vi "OldFieldToOOField.vi"(4 "Defense stretch":i32=500, 6 "Defense width":i32=1000, 8 "error in (no error)":errorcluster, 10 "geometry":T1, 11 "Field in":refnum<class "Field.lvclass">) -> (0 "error out":errorcluster, 3 "Field out":refnum<class "Field.lvclass">)   [LabVIEW 2023, in "Field.lvclass"]
uses:
  Field.lvclass
  Vision_class/Old vision/SSL Detection Frame Simple Estimator Cameras VelCmd Folder/Core/Field Size.ctl
  Field.lvclass/Field.ctl
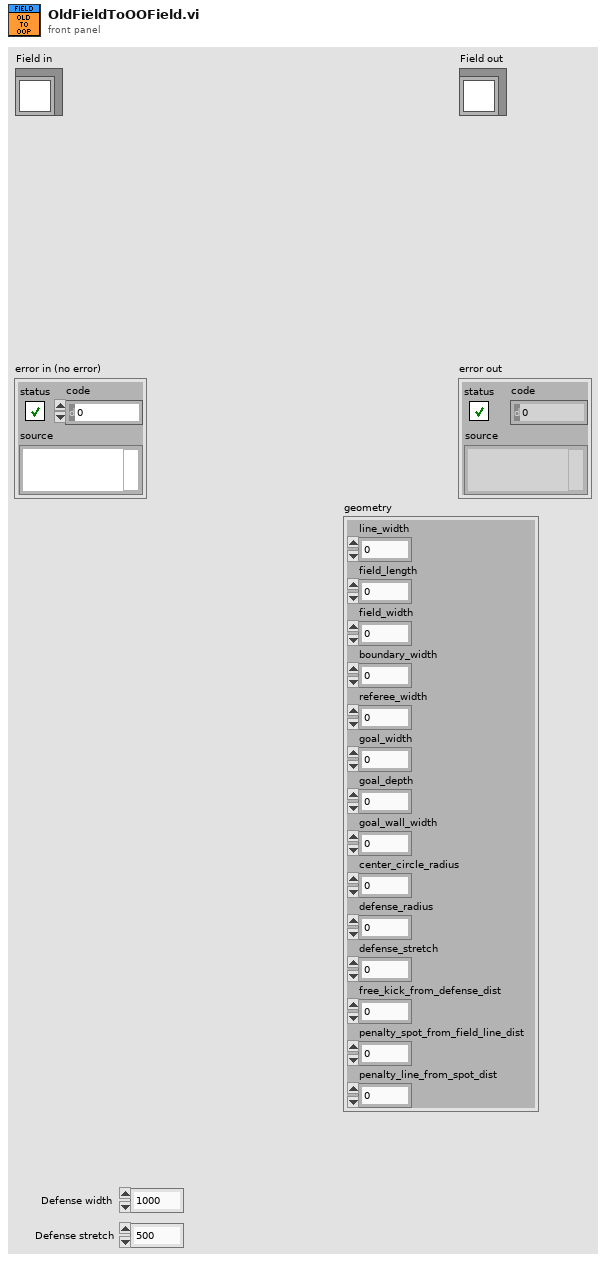
[diagram p1: front panel]
types:
  T1 = typedef "Field Size.ctl" = cluster{"line_width":u32, "field_length":u32, "field_width":u32, "boundary_width":u32, "referee_width":u32, "goal_width":u32, "goal_depth":u32, "goal_wall_width":u32, "center_circle_radius":u32, "defense_radius":u32, "defense_stretch":u32, "free_kick_from_defense_dist":u32, "penalty_spot_from_field_line_dist":u32, "penalty_line_from_spot_dist":u32}
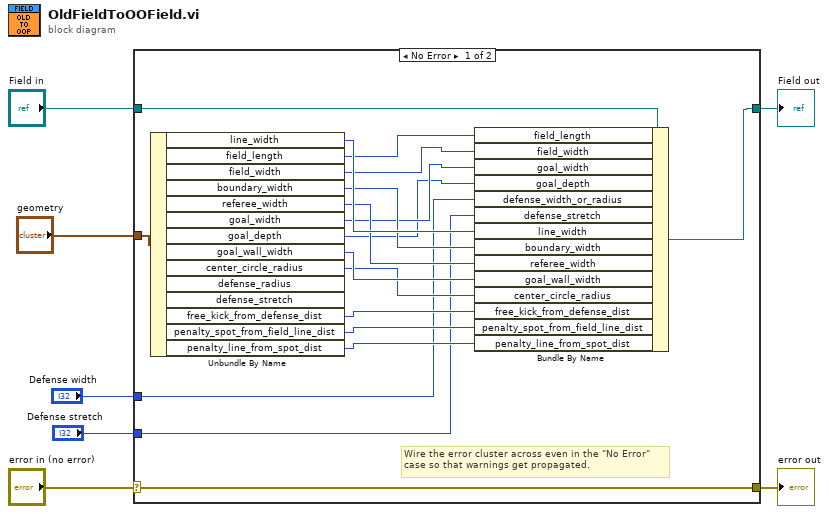
[diagram p0: block diagram]
diagram:
  n1 = case shown="No Error" "error in (no error)" {
    selector: "error in (no error)" -> [w25 w27]
    tunnel: [w25 w27] -> w6
    tunnel: [w10 w26] -> w4
    tunnel: "Field in" -> [w24 w26]
    tunnel: "geometry" -> [w23 _]
    tunnel: "Defense width" -> [w9 _]
    tunnel: "Defense stretch" -> [w8 _]
    frame No Error {
      # "Wire the error cluster across even in the \"No Error\"\ncase so that warnings get propagated."
      n2 = Unbundle By Name(w23) -> ("line_width"=w22:u32, "field_length"=w21:u32, "field_width"=w20:u32, "boundary_width"=w19:u32, "referee_width"=w18:u32, "goal_width"=w17:u32, "goal_depth"=w16:u32, "goal_wall_width"=w15:u32, "center_circle_radius"=w14:u32, "free_kick_from_defense_dist"=w13:u32, "penalty_spot_from_field_line_dist"=w12:u32, "penalty_line_from_spot_dist"=w11:u32)  [unwired: 2 out]
      n3 = Bundle By Name(cluster=w24, "field_length"=w21, "field_width"=w20, "goal_width"=w17, "goal_depth"=w16, "defense_width_or_radius"=w9, "defense_stretch"=w8, "line_width"=w22, "boundary_width"=w19, "referee_width"=w18, "goal_wall_width"=w15, "center_circle_radius"=w14, "free_kick_from_defense_dist"=w13, "penalty_spot_from_field_line_dist"=w12, "penalty_line_from_spot_dist"=w11) -> (w10:refnum<class "Field.lvclass">)
    }
    frame Error {
    }
  }
  "error out" <- w6
  "Field out" <- w4
